vi "Set_HTML_Data_NetRef.vi"(8 "error in (no error)":errorcluster, 10 "String":string="<!DOCTYPE HTML PUBLIC \"-//W3C//DTD HTML 4.01 Transitional//EN\">\n<html>\n  <head>\n\n    <meta http-equiv=\"content-type\" content=\"text/html; charset=UTF-8\">\n    <title>median_filter</title>\n  </head>\n  <body>\n    <h1 align=\"center\"><font color=\"#ff0000\"><b>CerberoII<font size=\"+3\"><sup>®</sup></font>\n          HELP</b></font></h1>\n    <h2 align=\"center\"><font color=\"#3333ff\">ME</font><font\n        color=\"#3333ff\">DIAN FILTER</font></h2>\n    <div align=\"center\"><img\nsrc=\"file:///C:/Users/Marco Preziani/Documents/Help_Crypting_repository/UserManual_FAR/filters/median_filter.PNG\"\n        alt=\"median_filter\" width=\"335\" height=\"201\"><br>\n      <br>\n    </div>\n    <p>In this window you can choose the parameters to set a median\n      filter:<br>\n    </p>\n    <ul>\n      <li>left rank: set the number of samples to use at the left side\n        of the sample to filter;\n      </li>\n      <li>right rank: set the number of samples to use at the right side\n        of the sample to filter;\n      </li>\n      <li>low/high pass: you can select if the median has to be low pass\n        or high pass;</li>\n    </ul>\n    <p>Note: the rank number cannot be higher than the packet number of\n      elements. <br>\n    </p>\n  </body>\n</html>\n", 11 "Folder_Mgmt in":refnum<class "WebBrowser_Mgmt.lvclass">) -> (0 "error out":errorcluster, 3 "Folder_Mgmt out":refnum<class "WebBrowser_Mgmt.lvclass">)   [LabVIEW 2016, in "WebBrowser_Mgmt.lvclass"]
uses:
  WebBrowser_Mgmt.lvclass
  WebBrowser_Mgmt.lvclass/WebBrowser_Mgmt.ctl
  System.Windows.Forms
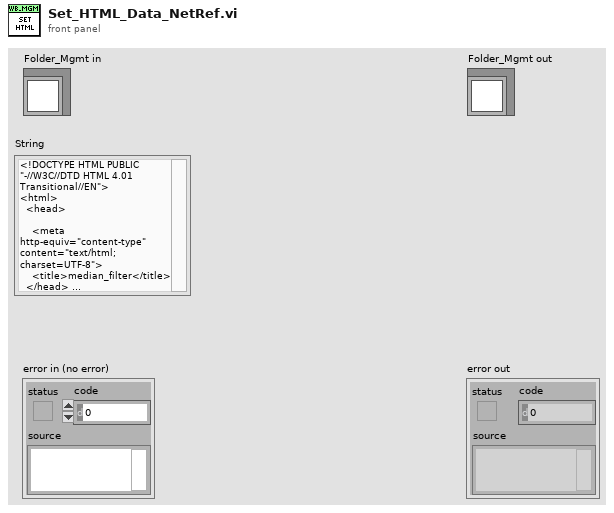
[diagram p1: front panel]
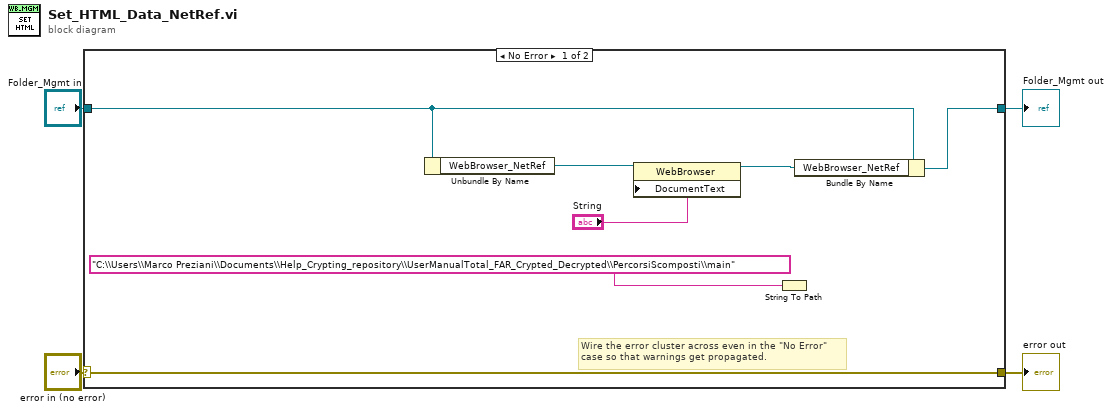
[diagram p0: block diagram]
diagram:
  n1 = case shown="No Error" "error in (no error)" {
    selector: "error in (no error)" -> [w11 w13]
    tunnel: [w11 w13] -> w3
    tunnel: [w7 w12] -> w1
    tunnel: "Folder_Mgmt in" -> [w8 w12]
    frame No Error {
      # "Wire the error cluster across even in the \"No Error\"\ncase so that warnings get propagated."
      n2 = Unbundle By Name(w8) -> ("WebBrowser_NetRef"=w9:refnum<k24>)
      n3 = property class="WebBrowser"(reference=w9, "DocumentText"="String") -> (reference out=w6:refnum<k24>)  [unwired: 1 in, 1 out]
      n4 = String To Path(string="C:\\Users\\Marco Preziani\\Documents\\Help_Crypting_repository\\UserManualTotal_FAR_Crypted_Decrypted\\PercorsiScomposti\\main" ("Domain")) -> ()  [unwired: 1 out]
      n5 = Bundle By Name(cluster=w8, "WebBrowser_NetRef"=w6) -> (w7:refnum<class "WebBrowser_Mgmt.lvclass">)
    }
    frame Error {
    }
  }
  "error out" <- w3
  "Folder_Mgmt out" <- w1
